vi "DELTA.vi"() -> ()   [LabVIEW 2013]
uses:
  <vilib>/LabVIEW Interface for Arduino/Type Defs/Pin Mode.ctl
  <vilib>/imath/engines/lvmath2/RunTimeEngine/NodeEndStatement/NIMS_NodeEndStatement_Output.vi
  <instcachedir>/0/NIMS_NodeEndStatement_Output_53EC0D466D134D7ABD903AC30B43404B.lvgen/NIMS_NodeEndStatement_Output_53EC0D466D134D7ABD903AC30B43404B_009.vi
  <vilib>/imath/engines/lvmath2/RunTimeEngine/BuiltInFunctions/atan/NIMS_atan(C).vi
  <instcachedir>/0/NIMS_atan(C)_7C2C2596D2F04E9E823B85B74D765718.lvgen/NIMS_atan(C)_7C2C2596D2F04E9E823B85B74D765718_001.vi
  <vilib>/imath/engines/lvmath2/RunTimeEngine/ErrorHandling/NIMS_Finalize Error.vi
  <vilib>/LabVIEW Interface for Arduino/LabVIEW Interface for Arduino.lvlib
panel:
  out "Reached 3":bool
  out "Reached 2":bool
  out "Reached 1":bool
  out "ESTADO":bool
  in  "HOME":bool
  out "Consigna Pinza":dbl(knob) scale=0.0..100.0
  in  "Abrir/Cerrar":bool
  out "Motor 3":dbl(knob) scale=-50.0..100.0
  out "Motor 2":dbl(knob) scale=-50.0..100.0
  out "Motor 1":dbl(knob) scale=-50.0..100.0
  in  "Z":dbl=-158.0 min=-320.0 max=-158.0
  in  "Y":dbl min=-80.0 max=80.0
  in  "X":dbl min=-80.0 max=80.0
  out "Potenciómetro 1":dbl(knob) scale=0.0..5.0
  out "Potenciómetro 2":dbl(knob) scale=0.0..5.0
  out "Potenciómetro 3":dbl(knob) scale=0.0..5.0
  out "Pinza":dbl(knob) scale=0.0..100.0
  in  "STOP":bool
  # "Panel de control de posición del Robot DELTA\n\nEl LED ESTADO del sistema indica si éste está operativo\no no. Por favor, espere a que se ilumine antes de usarlo.\n\nGracias."
  # "CINEMÁTICA INVERSA"
  # "CONSIGNAS"
  # "POSICIÓN MOTORES"
  # "CONTROL DE POSICIÓN DEL EFECTOR"
  # "Con los parámetros X, Y, Z de este panel se\nestablece la posición del centro del efector \nque se desea. Se limita la zona de actuación\na los valores aquí establecidos."
  # "Xmín = -80"
  # "Ymín = -80 mm"
  # "Zmín = -320"
  # "Xmáx = 80 mm"
  # "Ymáx = 80 mm"
  # "Zmáx = -158"
  # "PINZA"
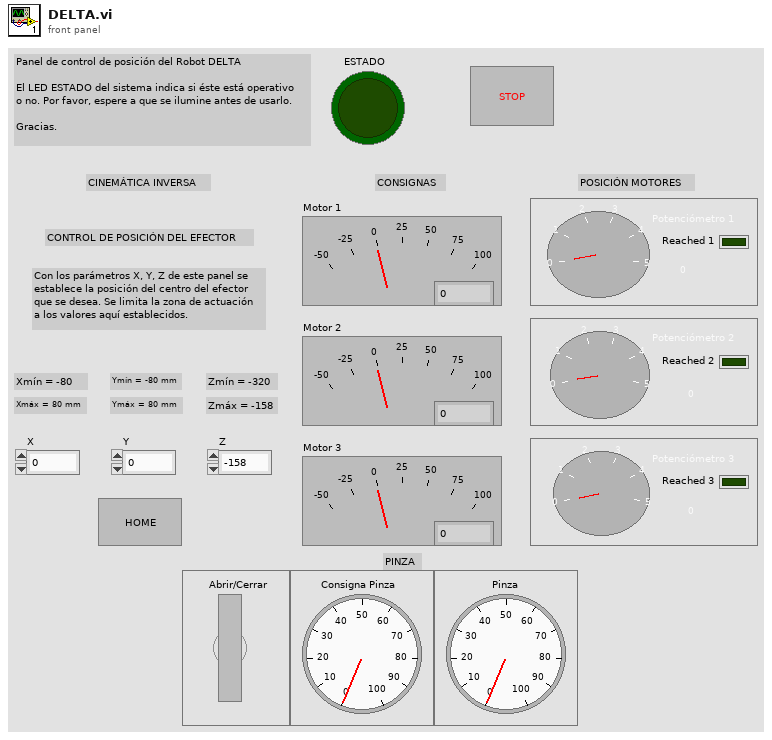
[diagram p1: front panel]
types:
  T1 = typedef "LabVIEW Interface for Arduino.lvlib/Pin Mode.ctl" = enum8{"Input", "Output"}
  T2 = typedef "LabVIEW Interface for Arduino.lvlib/Arduino Resource.ctl" = cluster{"VISA resource":refnum<visa-resource-name>, "Board Type":T3, "Connection Type":enum8{"USB / Serial"}, "Bytes Per Packet (15)":u8}
  T3 = typedef "LabVIEW Interface for Arduino.lvlib/Board Type.ctl" = enum16{"Uno", "Dimuelanove w/Atmega 328", "Mega 2560"}
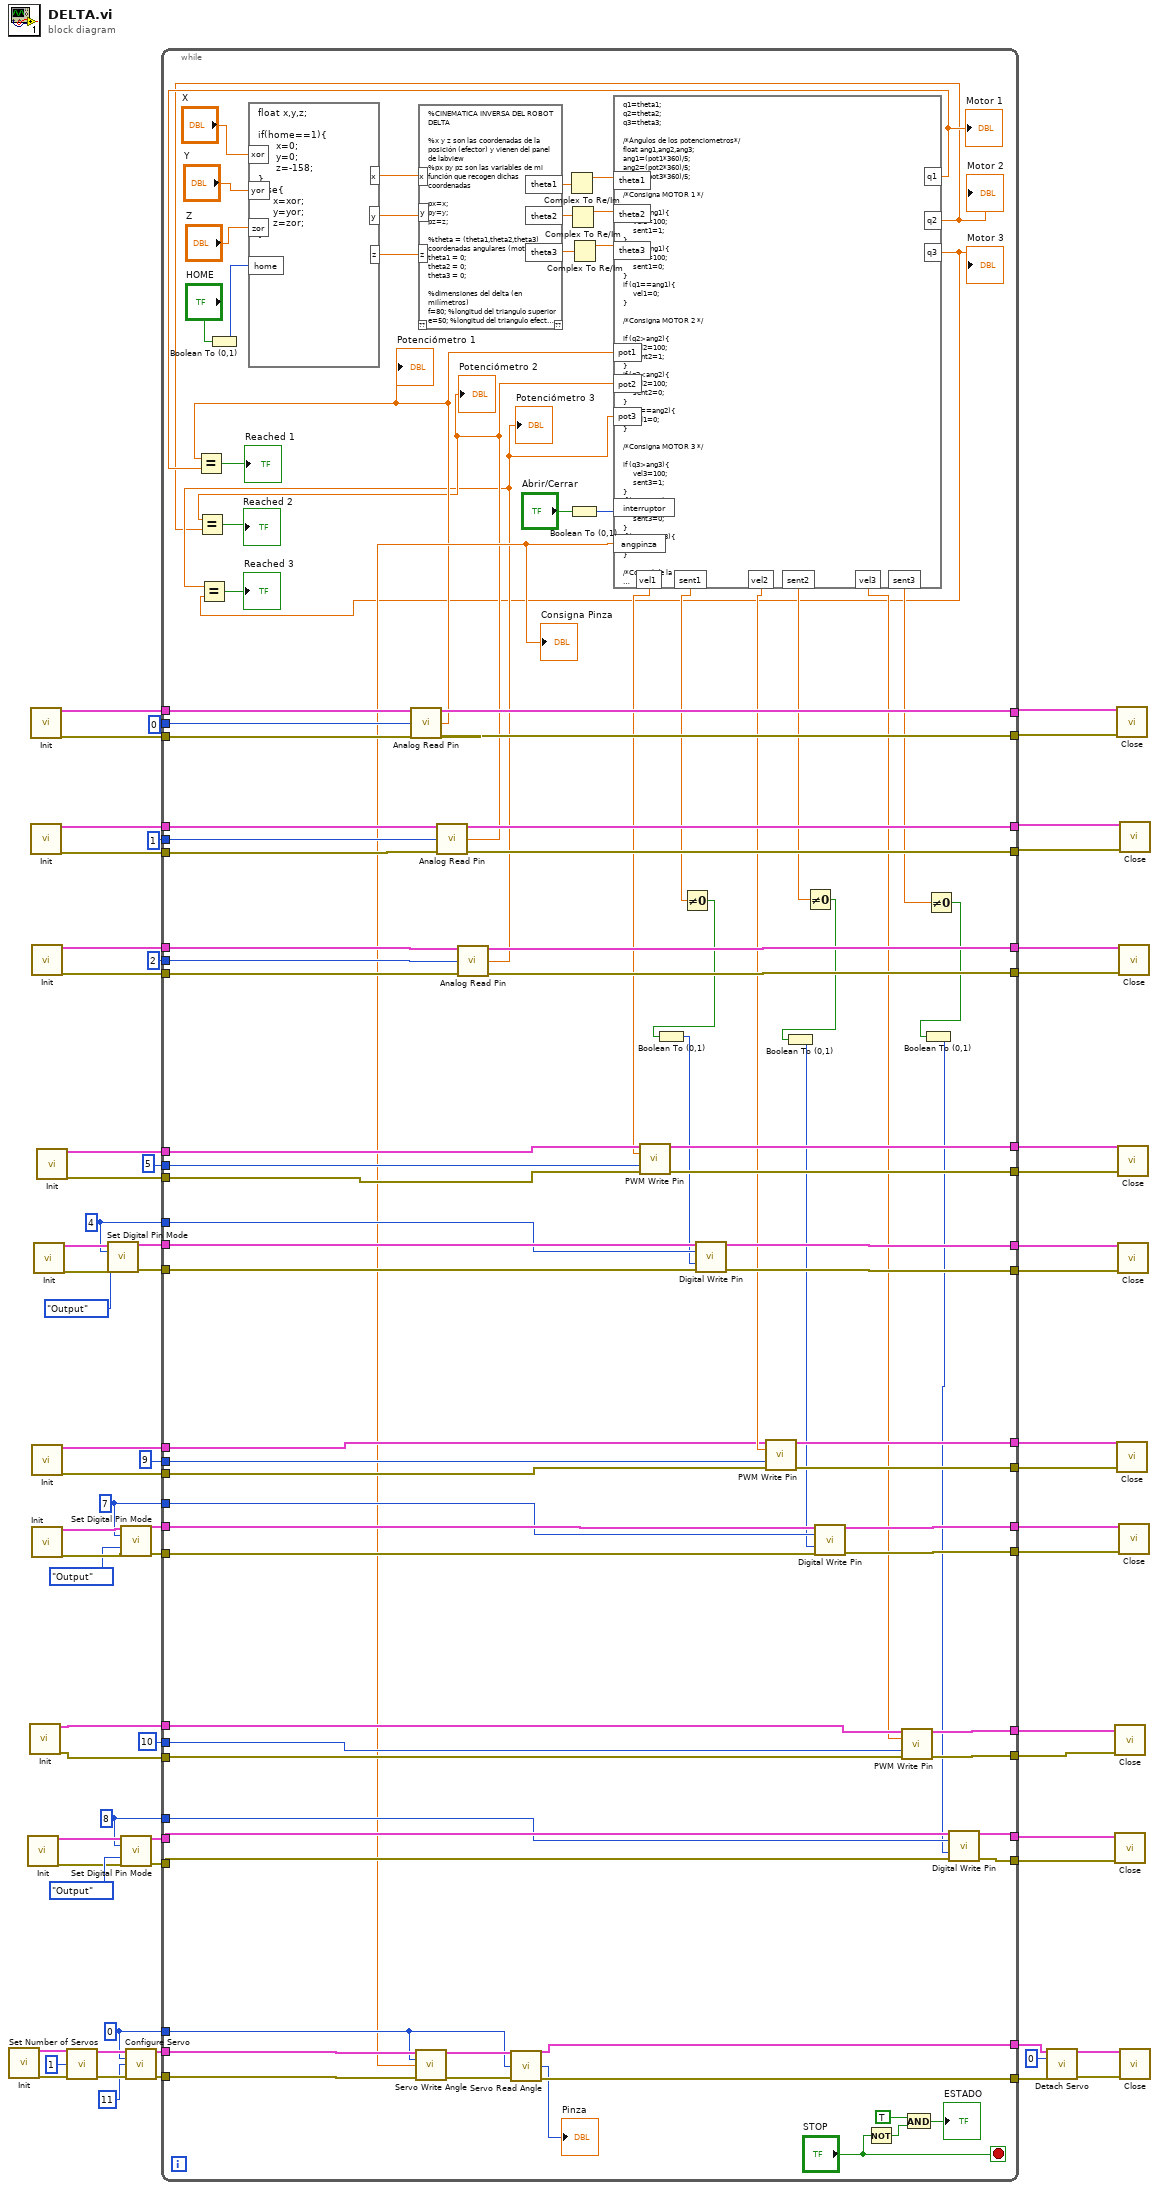
[diagram p0: block diagram]
diagram:
  w4 = u8 8 ("Digital I/O Pin")
  w12 = u8 7 ("Digital I/O Pin")
  w20 = u8 4 ("Digital I/O Pin")
  w60 = u8 0 ("Servo Number (0)")
  n1 = call <vilib>:"Init.vi"() -> ("Arduino Resource"=w68:T2, "error out"=w67:errorcluster)  [unwired: 18 in]
  n2 = call <vilib>:"Init.vi"() -> ("Arduino Resource"=w9:T2, "error out"=w7:errorcluster)  [unwired: 18 in]
  n3 = call <vilib>:"Init.vi"() -> ("Arduino Resource"=w46:T2, "error out"=w45:errorcluster)  [unwired: 18 in]
  n4 = call <vilib>:"Init.vi"() -> ("Arduino Resource"=w30:T2, "error out"=w29:errorcluster)  [unwired: 18 in]
  n5 = call <vilib>:"Init.vi"() -> ("Arduino Resource"=w35:T2, "error out"=w34:errorcluster)  [unwired: 18 in]
  n6 = call <vilib>:"Init.vi"() -> ("Arduino Resource"=w43:T2, "error out"=w42:errorcluster)  [unwired: 18 in]
  n7 = call <vilib>:"Init.vi"() -> ("Arduino Resource"=w50:T2, "error out"=w49:errorcluster)  [unwired: 18 in]
  n8 = call <vilib>:"Init.vi"() -> ("Arduino Resource"=w17:T2, "error out"=w16:errorcluster)  [unwired: 18 in]
  n9 = call <vilib>:"Init.vi"() -> ("Arduino Resource"=w24:T2, "error out"=w23:errorcluster)  [unwired: 18 in]
  n10 = call <vilib>:"Init.vi"() -> ("Arduino Resource"=w54:T2, "error out"=w53:errorcluster)  [unwired: 18 in]
  n11 = call <vilib>:"Set Number of Servos.vi"("Arduino Resource"=w68, "Number Of Servos (1)"=u8 1, "error in"=w67) -> ("Arduino Resource"=w65:T2, "error out"=w64:errorcluster)  [unwired: 11 in]
  n12 = call <vilib>:"Set Digital Pin Mode.vi"("Arduino Resource"=w24, "Digital I/O Pin"=w20, "Pin Mode (Input)"=Pin_Mode."Output", "error in"=w23) -> ("Arduino Resource"=w22:T2, "error out"=w21:errorcluster)  [unwired: 10 in]
  n13 = call <vilib>:"Set Digital Pin Mode.vi"("Arduino Resource"=w17, "Digital I/O Pin"=w12, "Pin Mode (Input)"=Pin_Mode."Output", "error in"=w16) -> ("Arduino Resource"=w14:T2, "error out"=w13:errorcluster)  [unwired: 10 in]
  n14 = call <vilib>:"Set Digital Pin Mode.vi"("Arduino Resource"=w9, "Digital I/O Pin"=w4, "Pin Mode (Input)"=Pin_Mode."Output", "error in"=w7) -> ("Arduino Resource"=w6:T2, "error out"=w5:errorcluster)  [unwired: 10 in]
  n15 = call <vilib>:"Configure Servo.vi"("Arduino Resource"=w65, "Servo Number (0)"=w60, "DIO Pin (2)"=u8 11, "error in"=w64) -> ("Arduino Resource"=w62:T2, "error out"=w61:errorcluster)  [unwired: 10 in]
  n16 = while {
    tunnel: w62 -> [w163]
    tunnel: w61 -> [w162]
    tunnel: w60 -> [w159]
    tunnel: [w158] -> w58
    tunnel: [w157] -> w57
    tunnel: w54 -> [w155]
    tunnel: w53 -> [w154]
    tunnel: [w153] -> w52
    tunnel: [w152] -> w51
    tunnel: w50 -> [w104]
    tunnel: w49 -> [w151]
    tunnel: [w150] -> w48
    tunnel: [w149] -> w47
    tunnel: w46 -> [w100]
    tunnel: w45 -> [w99]
    tunnel: [w148] -> w44
    tunnel: w43 -> [w145]
    tunnel: w42 -> [w144]
    tunnel: u8 5 ("PWM Pin (3)") -> [w147]
    tunnel: u8 9 ("PWM Pin (3)") -> [w146]
    tunnel: u8 10 ("PWM Pin (3)") -> [w98]
    tunnel: u8 2 ("Analog Input Pin (0)") -> [w143]
    tunnel: [w142] -> w37
    tunnel: [w141] -> w36
    tunnel: w35 -> [w140]
    tunnel: w34 -> [w139]
    tunnel: u8 1 ("Analog Input Pin (0)") -> [w138]
    tunnel: [w137] -> w32
    tunnel: [w136] -> w31
    tunnel: w30 -> [w135]
    tunnel: w29 -> [w134]
    tunnel: [w133] -> w27
    tunnel: [w132] -> w26
    tunnel: u8 0 ("Analog Input Pin (0)") -> [w131]
    tunnel: w22 -> [w130]
    tunnel: w21 -> [w129]
    tunnel: w20 -> [w128]
    tunnel: [w127] -> w19
    tunnel: [w126] -> w18
    tunnel: w14 -> [w125]
    tunnel: w13 -> [w124]
    tunnel: w12 -> [w123]
    tunnel: [w122] -> w11
    tunnel: [w121] -> w10
    tunnel: w6 -> [w120]
    tunnel: w5 -> [w119]
    tunnel: w4 -> [w118]
    tunnel: [w117] -> w3
    tunnel: [w116] -> w2
    tunnel: [w96] -> w1
    stop <- "STOP" stop-if-true
    n17 = Boolean To (0,1)(Boolean="HOME") -> (0, 1=w85:i16)
    n18 = formula code="float x,y,z;\n\nif(home==1){\n      x=0;\n      y=0;\n      z=-158;\n}\nelse{\n     x=xor;\n     y=yor;\n     z=zor;\n}"("xor"="X", "yor"="Y", "zor"="Z", "home"=w85) -> ("x"=w83:dbl, "y"=w84:dbl, "z"=w82:dbl)
    n19 = call <vilib>:"Analog Read Pin.vi"("Arduino Resource"=w135, "Analog Input Pin (0)"=w131, "error in"=w134) -> ("Arduino Resource"=w133:T2, "Voltage"=w74:dbl, "error out"=w132:errorcluster)  [unwired: 10 in]
    "Potenciómetro 1" <- w74
    n20 = mathscript code="%CINEMATICA INVERSA DEL ROBOT DELTA\n\n%x y z son las coordenadas de la posición (efector) y vienen del panel de labview\n%px py pz son las variables de mi función que recogen dichas coordenadas\n\npx=x;\npy=y;\npz=z;\n\n%theta = (theta1,theta2,theta3) coordenadas angulares (motores)\ntheta1 = 0;\ntheta2 = 0;\ntheta3 = 0;\n\n%dimensiones del delta (en milímetros)\nf=80; %longitud del triangulo superior\ne=50; %longitud del triangulo efector\nrf=110; %longitud de los ejes superiores\nre=240; %longitud de los ejes inferiores\n\n\n%calculamos la coordenada articular theta1 que será mi consigna\npy1=-f/2*tan(pi/6);\npy=py-0.5*0.57735*e;\n%calculo los coeficientes a y b de la ecuacion z=a+b*y\na=(px*px+py*py+pz*pz+rf*rf-re*re-py1*py1)/(2*pz);\nb=(py1-py)/pz;\n%calculo el discriminante para saber si el punto es alcanzable\nd=-(a+b*py1)*(a+b*py1)+rf*(b*b*rf+rf);\nif d>0 %si el discriminante es positivo, el punto es alcanzable\n    pyj=(py1-a*b-sqrt(d))/(b*b+1); %resolución de la ecuación cuadrática\n    pzj=a+b*pyj; %aplicamos la ecuacion z=a+b*y a los puntos auxiliares calculados\n    if pyj>py1\n        theta1=180*atan(-pzj/(py1-pyj))/pi+180;\n    else\n        theta1=180*atan(-pzj/(py1-pyj))/pi;\n    end\n        \nelse %si el discriminante es negativo, el punto no es alcanzable\n    theta1=0;\nend\n\n%repetimos el proceso para el segundo motor\n%proyectamos las coordenadas\npx=x*cos(120*pi/180)+y*sin(120*pi/180);\npy=y*cos(120*pi/180)-x*sin(120*pi/180);\npz=z;\n\n%calculamos la coordenada articular theta2 que será mi consigna\npy1=-f/2*tan(pi/6);\npy=py-0.5*0.57735*e;\n%calculo los coeficientes a y b de la ecuacion z=a+b*y\na=(px*px+py*py+pz*pz+rf*rf-re*re-py1*py1)/(2*pz);\nb=(py1-py)/pz;\n%calculo el discriminante para saber si el punto es alcanzable\nd=-(a+b*py1)*(a+b*py1)+rf*(b*b*rf+rf);\nif d>0 %si el discriminante es positivo, el punto es alcanzable\n    pyj=(py1-a*b-sqrt(d))/(b*b+1); %resolución de la ecuación cuadrática\n    pzj=a+b*pyj; %aplicamos la ecuacion z=a+b*y a los puntos auxiliares calculados\n    if pyj>py1\n        theta2=180*atan(-pzj/(py1-pyj))/pi+180;\n    else\n        theta2=180*atan(-pzj/(py1-pyj))/pi;\n    end\n        \nelse %si el discriminante es negativo, el punto no es alcanzable\n    theta2=0;\nend\n\n%repetimos el proceso para el tercer motor\n%proyectamos las coordenadas\npx=x*cos(120*pi/180)-y*sin(120*pi/180);\npy=y*cos(120*pi/180)+x*sin(120*pi/180);\npz=z;\n\n%calculamos la coordenada articular theta3 que será mi consigna\npy1=-f/2*tan(pi/6);\npy=py-0.5*0.57735*e;\n%calculo los coeficientes a y b de la ecuacion z=a+b*y\na=(px*px+py*py+pz*pz+rf*rf-re*re-py1*py1)/(2*pz);\nb=(py1-py)/pz;\n%calculo el discriminante para saber si el punto es alcanzable\nd=-(a+b*py1)*(a+b*py1)+rf*(b*b*rf+rf);\nif d>0 %si el discriminante es positivo, el punto es alcanzable\n    pyj=(py1-a*b-sqrt(d))/(b*b+1); %resolución de la ecuación cuadrática\n    pzj=a+b*pyj; %aplicamos la ecuacion z=a+b*y a los puntos auxiliares calculados\n    if pyj>py1\n        theta3=180*atan(-pzj/(py1-pyj))/pi+180;\n    else\n        theta3=180*atan(-pzj/(py1-pyj))/pi;\n    end\n        \nelse %si el discriminante es negativo, el punto no es alcanzable\n    theta3=0;\nend\n\n%Ya tenemos nuestras coordenadas angulares para las x,y,z dadas\ntheta=[theta1,theta2,theta3];"("x"=w83, "y"=w84, "z"=w82) -> ("theta1"=w115:cdb, "theta2"=w113:cdb, "theta3"=w111:cdb)  [unwired: 1 in, 1 out]
    n21 = call <vilib>:"Analog Read Pin.vi"("Arduino Resource"=w140, "Analog Input Pin (0)"=w138, "error in"=w139) -> ("Arduino Resource"=w137:T2, "Voltage"=w73:dbl, "error out"=w136:errorcluster)  [unwired: 10 in]
    "Potenciómetro 2" <- w73
    n22 = call <vilib>:"Analog Read Pin.vi"("Arduino Resource"=w145, "Analog Input Pin (0)"=w143, "error in"=w144) -> ("Arduino Resource"=w142:T2, "Voltage"=w72:dbl, "error out"=w141:errorcluster)  [unwired: 10 in]
    "Potenciómetro 3" <- w72
    n23 = Complex To Re/Im(x + iy=w115) -> (x=w114:dbl)  [unwired: 1 out]
    n24 = Complex To Re/Im(x + iy=w113) -> (x=w112:dbl)  [unwired: 1 out]
    n25 = Boolean To (0,1)(Boolean="Abrir/Cerrar") -> (0, 1=w91:i16)
    n26 = Complex To Re/Im(x + iy=w111) -> (x=w110:dbl)  [unwired: 1 out]
    n27 = formula code="q1=theta1;\nq2=theta2;\nq3=theta3;\n\n/*Ángulos de los potenciometros*/\nfloat ang1,ang2,ang3;\nang1=(pot1*360)/5;\nang2=(pot2*360)/5;\nang3=(pot3*360)/5;\n\n/*Consigna MOTOR 1 */\n\nif (q1>ang1){\n     vel1=100;\n     sent1=1;\n}\nif (q1<ang1){\n     vel1=100;\n     sent1=0;\n}\nif (q1==ang1){\n     vel1=0;\n}\n\n/*Consigna MOTOR 2 */\n\nif (q2>ang2){\n     vel2=100;\n     sent2=1;\n}\nif (q2<ang2){\n     vel2=100;\n     sent2=0;\n}\nif (q2==ang2){\n     vel1=0;\n}\n\n/*Consigna MOTOR 3 */\n\nif (q3>ang3){\n     vel3=100;\n     sent3=1;\n}\nif (q3<ang3){\n     vel3=100;\n     sent3=0;\n}\nif (q3==ang3){\n     vel3=0;\n}\n\n/*Control de la pinza*/\n\nif (interruptor==1){\n     angpinza=0;\n}\nif (interruptor==0){\n     angpinza=100;\n}"("theta1"=w114, "theta2"=w112, "theta3"=w110, "pot1"=w74, "pot2"=w73, "pot3"=w72, "interruptor"=w91) -> ("q1"=w71:dbl, "q2"=w70:dbl, "q3"=w69:dbl, "vel1"=w109:dbl, "sent1"=w108:dbl, "vel2"=w105:dbl, "sent2"=w102:dbl, "vel3"=w97:dbl, "sent3"=w93:dbl, "angpinza"=w90:dbl)
    "Motor 1" <- w71
    "Motor 2" <- w70
    "Motor 3" <- w69
    "Consigna Pinza" <- w90
    n28 = Equal?(x=w74, y=w71) -> (x = y?=→"Reached 1":bool)
    n29 = Equal?(x=w73, y=w70) -> (x = y?=→"Reached 2":bool)
    n30 = Equal?(x=w72, y=w69) -> (x = y?=→"Reached 3":bool)
    n31 = call <vilib>:"Servo Write Angle.vi"("Arduino Resource"=w163, "Servo Number"=w159, "Angle (Degrees)"=w90, "error in"=w162) -> ("Arduino Resource"=w161:T2, "error out"=w160:errorcluster)  [unwired: 10 in]
    n32 = call <vilib>:"Servo Read Angle.vi"("Arduino Resource"=w161, "Servo Number"=w159, "error in"=w160) -> ("Arduino Resource"=w158:T2, "Angle (Degrees)"=→"Pinza":u8, "error out"=w157:errorcluster)  [unwired: 10 in]
    n33 = call <vilib>:"PWM Write Pin.vi"("Arduino Resource"=w155, "Duty Cycle (0 - 255)"=w109, "PWM Pin (3)"=w147, "error in"=w154) -> ("Arduino Resource"=w153:T2, "error out"=w152:errorcluster)  [unwired: 10 in]
    n34 = Not Equal To 0?(x=w108) -> (x != 0?=w107:bool)
    n35 = Boolean To (0,1)(Boolean=w107) -> (0, 1=w106:i16)
    n36 = call <vilib>:"Digital Write Pin.vi"("Arduino Resource"=w130, "Digital I/O Pin (0)"=w128, "Value (0)"=w106, "error in"=w129) -> ("Arduino Resource"=w127:T2, "error out"=w126:errorcluster)  [unwired: 10 in]
    n37 = call <vilib>:"PWM Write Pin.vi"("Arduino Resource"=w104, "Duty Cycle (0 - 255)"=w105, "PWM Pin (3)"=w146, "error in"=w151) -> ("Arduino Resource"=w150:T2, "error out"=w149:errorcluster)  [unwired: 10 in]
    n38 = Not Equal To 0?(x=w102) -> (x != 0?=w103:bool)
    n39 = Boolean To (0,1)(Boolean=w103) -> (0, 1=w101:i16)
    n40 = call <vilib>:"Digital Write Pin.vi"("Arduino Resource"=w125, "Digital I/O Pin (0)"=w123, "Value (0)"=w101, "error in"=w124) -> ("Arduino Resource"=w122:T2, "error out"=w121:errorcluster)  [unwired: 10 in]
    n41 = Not(x="STOP") -> (.not. x?=w80:bool)
    n42 = call <vilib>:"PWM Write Pin.vi"("Arduino Resource"=w100, "Duty Cycle (0 - 255)"=w97, "PWM Pin (3)"=w98, "error in"=w99) -> ("Arduino Resource"=w96:T2, "error out"=w148:errorcluster)  [unwired: 10 in]
    n43 = And(x=TRUE, y=w80) -> (x .and. y?=→"ESTADO":bool)
    n44 = Not Equal To 0?(x=w93) -> (x != 0?=w95:bool)
    n45 = Boolean To (0,1)(Boolean=w95) -> (0, 1=w94:i16)
    n46 = call <vilib>:"Digital Write Pin.vi"("Arduino Resource"=w120, "Digital I/O Pin (0)"=w118, "Value (0)"=w94, "error in"=w119) -> ("Arduino Resource"=w117:T2, "error out"=w116:errorcluster)  [unwired: 10 in]
  }
  n47 = call <vilib>:"Detach Servo.vi"("Arduino Resource"=w58, "Servo Number"=u8 0, "error in"=w57) -> ("Arduino Resource"=w56:T2, "error out"=w55:errorcluster)  [unwired: 11 in]
  n48 = call <vilib>:"Close.vi"("Arduino Resource"=w1, "error in"=w44) -> ()  [unwired: 13 in, 1 out]
  n49 = call <vilib>:"Close.vi"("Arduino Resource"=w3, "error in"=w2) -> ()  [unwired: 13 in, 1 out]
  n50 = call <vilib>:"Close.vi"("Arduino Resource"=w27, "error in"=w26) -> ()  [unwired: 13 in, 1 out]
  n51 = call <vilib>:"Close.vi"("Arduino Resource"=w48, "error in"=w47) -> ()  [unwired: 13 in, 1 out]
  n52 = call <vilib>:"Close.vi"("Arduino Resource"=w52, "error in"=w51) -> ()  [unwired: 13 in, 1 out]
  n53 = call <vilib>:"Close.vi"("Arduino Resource"=w19, "error in"=w18) -> ()  [unwired: 13 in, 1 out]
  n54 = call <vilib>:"Close.vi"("Arduino Resource"=w37, "error in"=w36) -> ()  [unwired: 13 in, 1 out]
  n55 = call <vilib>:"Close.vi"("Arduino Resource"=w11, "error in"=w10) -> ()  [unwired: 13 in, 1 out]
  n56 = call <vilib>:"Close.vi"("Arduino Resource"=w32, "error in"=w31) -> ()  [unwired: 13 in, 1 out]
  n57 = call <vilib>:"Close.vi"("Arduino Resource"=w56, "error in"=w55) -> ()  [unwired: 13 in, 1 out]
